vi "Initialize.vi"(8 "Error In":errorcluster, 11 "CS++MessageLogger in":refnum<class "CS++MessageLogger.lvclass">) -> (0 "Error Out":errorcluster, 3 "CS++MessageLogger out":refnum<class "CS++MessageLogger.lvclass">)   [LabVIEW 2015, in "CS++BaseClasses.lvlib" / "CS++MessageLogger.lvclass"]
doc: "Initialize the message logger client."
uses:
  CS++MessageLogger.lvclass
  Libraries/Base/CS++Base.lvlib
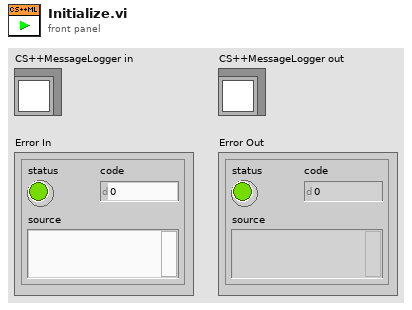
[diagram p1: front panel]
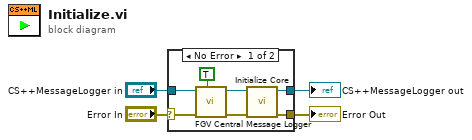
[diagram p0: block diagram]
diagram:
  n1 = case shown="No Error" "Error In" {
    selector: "Error In" -> [w9 w12]
    tunnel: [w8 w12] -> w3
    tunnel: [w10 w11] -> w1
    tunnel: "CS++MessageLogger in" -> [w7 w11]
    frame No Error {
      n2 = call "FGV Central Message Logger.vi"("Write? (F)"=TRUE, "CS++MessageLogger in"=w7) -> ("CS++MessageLogger out"=w6:refnum<class "CS++MessageLogger.lvclass">)  [unwired: 8 in, 1 out]
      n3 = call-dynamic "Initialize Core.vi"("Error In"=w9, "CS++MessageLogger in"=w6) -> ("Error Out"=w8:errorcluster, "CS++MessageLogger out"=w10:refnum<class "CS++MessageLogger.lvclass">)  [unwired: 8 in]
    }
    frame Error {
    }
  }
  "Error Out" <- w3
  "CS++MessageLogger out" <- w1
